vi "Sample Variance PtByPt.vi"(0 "x":dbl format="%0.2f", 1 "sample length":i32=100, 2 "initialize":bool) -> (3 "mean":dbl format="%0.2f", 4 "sample variance":dbl format="%0.2f", 5 "error":i32)   [LabVIEW 2020, in "NI_PtbyPt.lvlib"]
doc: "Computes the <B>mean</B> and <B>sample variance</B> of the values in the set of input data points specified by <B>sample length</B>."
uses:
  NI_PtbyPt.lvlib
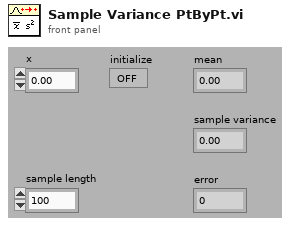
[diagram p1: front panel]
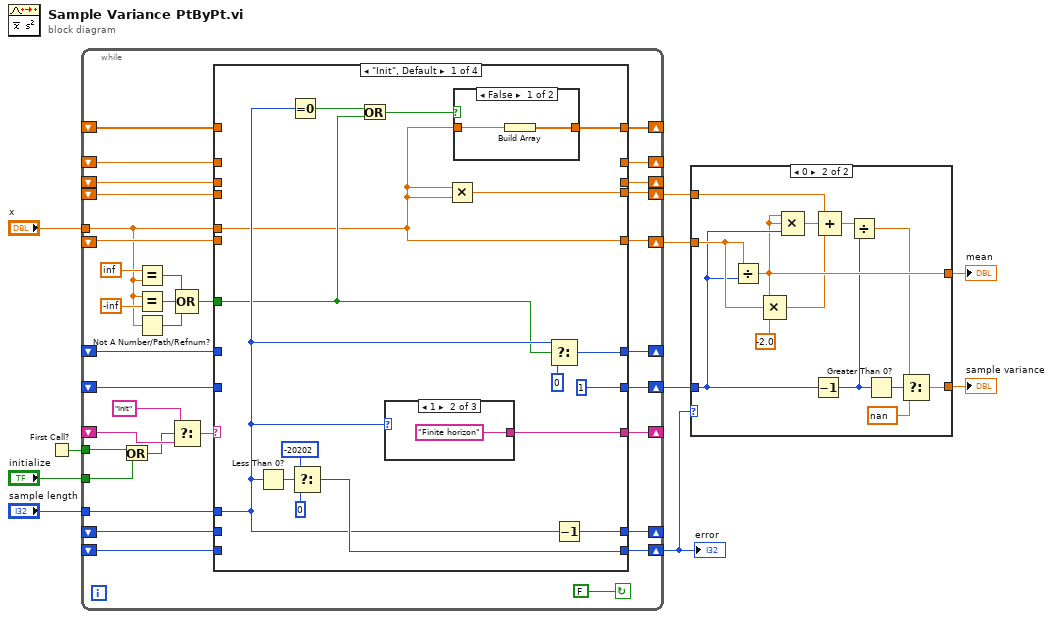
[diagram p0: block diagram]
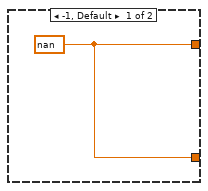
[diagram p2: hidden frame]
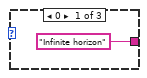
[diagram p4: hidden frame]
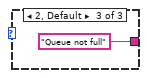
[diagram p5: hidden frame]
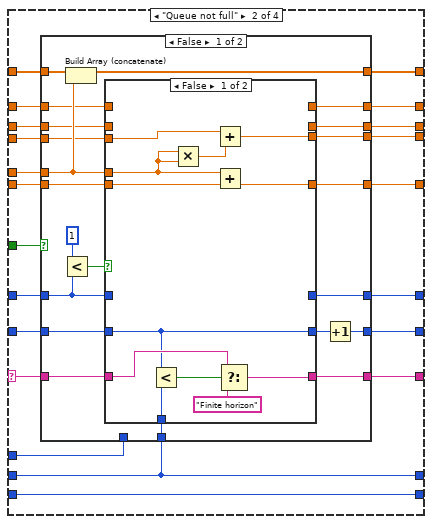
[diagram p6: hidden frame]
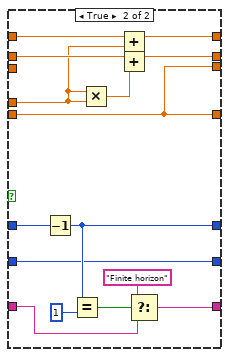
[diagram p7: hidden frame]
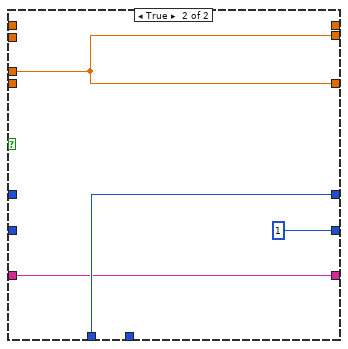
[diagram p8: hidden frame]
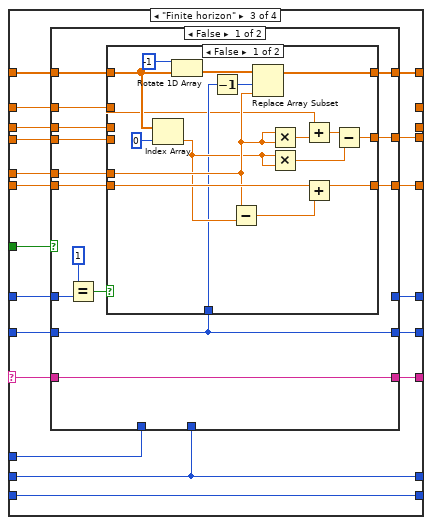
[diagram p9: hidden frame]
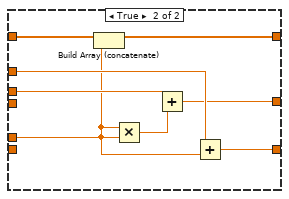
[diagram p10: hidden frame]
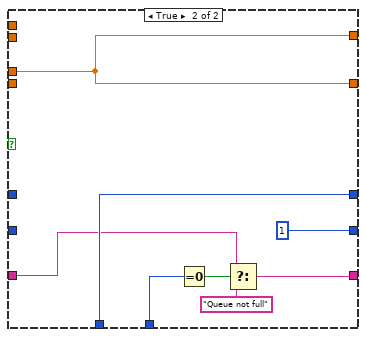
[diagram p11: hidden frame]
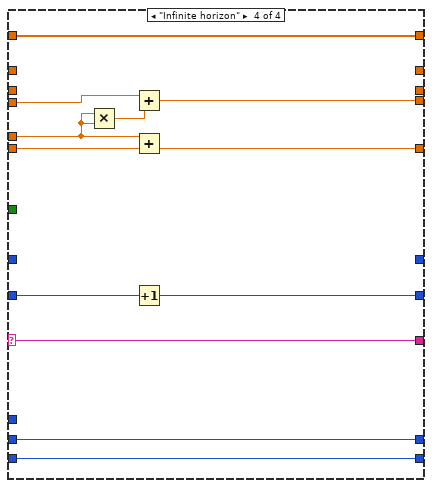
[diagram p12: hidden frame]
diagram:
  n1 = First Call?() -> (First Call?: T/F=w6:bool)
  n2 = while {
    tunnel: w6 -> [w29]
    shift-left: _ -> [w32]
    shift-right: [w31] -> _
    shift-left: _ -> [w33]
    shift-right: [w34] -> w9
    shift-left: _ -> [w36]
    shift-right: [w35] -> _
    shift-left: _ -> [w38]
    shift-right: [w39] -> w8
    shift-left: _ -> [w40]
    shift-right: [w41] -> w10
    shift-left: _ -> [w44]
    shift-right: [w37] -> _
    shift-right: [w21] -> _
    shift-left: _ -> [w16]
    shift-right: [w20] -> _
    shift-left: _ -> [w19]
    shift-right: [w18] -> _
    shift-left: _ -> [w17]
    shift-right: [w15] -> w5
    shift-left: _ -> [w14]
    tunnel: "x" -> [w13]
    tunnel: "sample length" -> [w12]
    tunnel: "initialize" -> [w11]
    stop <- FALSE continue-if-true
    n3 = Or(x=w29, y=w11) -> (x .or. y?=w28:bool)
    n4 = Equal?(x=inf, y=w13) -> (x = y?=w24:bool)
    n5 = Equal?(x=w13, y=-inf) -> (x = y?=w25:bool)
    n6 = Not A Number/Path/Refnum?(number/path/refnum=w13) -> (NaN/Path/Refnum?=w23:bool)
    n7 = Select(t="Init", s=w28, f=w44) -> (s? t:f=w42:string)
    n8 = Compound Arithmetic op=OR(w24, w25, w23) -> (w22:bool)
    n9 = case shown="\"Init\", Default" w42 {
      selector: w42 -> [_ w82 w149 w213]
      tunnel: [w45 w84 w154 w215] -> w41
      tunnel: w40 -> [_ w78 w151 w216]
      tunnel: w13 -> [w45 w80 w150 w209]
      tunnel: [1 w67 w147 w205] -> w39
      tunnel: w38 -> [_ w83 w157 w214]
      tunnel: [w51 w81 w148 w213] -> w37
      tunnel: w36 -> [_ w86 w155 w212]
      tunnel: [w46 w85 w156 w212] -> w35
      tunnel: w12 -> [w50 w68 w142 _]
      tunnel: [w56 w79 w152 w208] -> w34
      tunnel: w33 -> [_ w77 w153 w211]
      tunnel: [w55 w76 w140 w207] -> w31
      tunnel: w32 -> [_ w76 w140 w207]
      tunnel: w22 -> [w48 w75 w146 _]
      tunnel: [w53 w69 w141 _] -> w21
      tunnel: [_ w74 _ _] -> w20
      tunnel: w19 -> [_ w73 w143 _]
      tunnel: [_ w72 _ _] -> w18
      tunnel: w17 -> [_ w71 w144 _]
      tunnel: w16 -> [_ w70 w145 _]
      tunnel: [w52 w66 w139 w206] -> w15
      tunnel: w14 -> [_ w66 w139 w206]
      frame "Init", Default {
        n10 = Less Than 0?(x=w50) -> (x < 0?=w57:bool)
        n11 = Equal To 0?(x=w50) -> (x = 0?=w49:bool)
        n12 = Select(t=-20202, s=w57, f=0) -> (s? t:f=w52:i32)
        n13 = Or(x=w49, y=w48) -> (x .or. y?=w47:bool)
        n14 = case shown="1" w50 {
          tunnel: ["Infinite horizon" "Finite horizon" "Queue not full" ("f")] -> w51
          frame 0 {
          }
          frame 1 {
          }
          frame 2, Default {
          }
        }
        n15 = Multiply(x=w45, y=w45) -> (x*y=w56:dbl)
        n16 = case shown="False" w47 {
          tunnel: [w62 _] -> w46
          tunnel: w45 -> [w61 _]
          frame False {
            n17 = Build Array(w61) -> (w62:dbl[])
          }
          frame True {
          }
        }
        n18 = Select(t=w50, s=w48, f=0) -> (s? t:f=w53:i32)
        n19 = Decrement(x=w50) -> (x-1=w55:i32)
      }
      frame "Queue not full" {
        n20 = case shown="False" w75 {
          tunnel: w86 -> [w107 _]
          tunnel: [w106 _] -> w85
          tunnel: [w105 w135] -> w84
          tunnel: w83 -> [w97 _]
          tunnel: w82 -> [w104 w136]
          tunnel: [w103 w136] -> w81
          tunnel: w80 -> [w102 w135]
          tunnel: [w101 w135] -> w79
          tunnel: w78 -> [w100 _]
          tunnel: w77 -> [w99 _]
          tunnel: w76 -> [w98 _]
          tunnel: [w90 1] -> w67
          tunnel: [w95 _] -> w74
          tunnel: w73 -> [w94 _]
          tunnel: [w93 _] -> w72
          tunnel: w71 -> [w92 _]
          tunnel: w70 -> [w87 _]
          tunnel: [w91 w138] -> w69
          tunnel: w68 -> [_ w138]
          frame False {
            n21 = Less?(x=1, y=w87) -> (x < y?=w88:bool)
            n22 = Build Array (concatenate)(w107, w102) -> (w106:dbl[])
            n23 = case shown="False" w88 {
              tunnel: [w119 w128] -> w105
              tunnel: w104 -> [w117 w120]
              tunnel: [w115 w121] -> w103
              tunnel: w102 -> [w114 w131]
              tunnel: [w113 w128] -> w101
              tunnel: w100 -> [w112 w128]
              tunnel: w99 -> [w111 _]
              tunnel: w98 -> [w109 _]
              tunnel: w97 -> [w108 w122]
              tunnel: [w108 w122] -> w96
              tunnel: [_ w133] -> w95
              tunnel: w94 -> [_ w132]
              tunnel: [_ w130] -> w93
              tunnel: w92 -> [_ w129]
              tunnel: w87 -> [_ w124]
              tunnel: [_ w123] -> w91
              frame False {
                n24 = Less?(x=w108, y=w109) -> (x < y?=w118:bool)
                n25 = Multiply(x=w114, y=w114) -> (x*y=w110:dbl)
                n26 = Add(x=w111, y=w110) -> (x+y=w113:dbl)
                n27 = Add(x=w114, y=w112) -> (x+y=w119:dbl)
                n28 = Select(t=w117, s=w118, f="Finite horizon") -> (s? t:f=w115:string)
              }
              frame True {
                n29 = Decrement(x=w124) -> (x-1=w123:i32)
                n30 = Equal?(x=w123, y=1) -> (x = y?=w127:bool)
                n31 = Multiply(x=w131, y=w131) -> (x*y=w134:dbl)
                n32 = Add(x=w129, y=w131) -> (x+y=w130:dbl)
                n33 = Add(x=w132, y=w134) -> (x+y=w133:dbl)
                n34 = Select(t="Finite horizon" ("f"), s=w127, f=w120) -> (s? t:f=w121:string)
              }
            }
            n35 = Increment(x=w96) -> (x+1=w90:i32)
          }
          frame True {
          }
        }
      }
      frame "Finite horizon" {
        n36 = case shown="False" w146 {
          tunnel: w157 -> [w163 _]
          tunnel: [w171 _] -> w156
          tunnel: w155 -> [w170 _]
          tunnel: [w169 w197] -> w154
          tunnel: w153 -> [w168 _]
          tunnel: [w167 w197] -> w152
          tunnel: w151 -> [w166 _]
          tunnel: w150 -> [w165 w197]
          tunnel: w149 -> [w164 w198]
          tunnel: [w164 w200] -> w148
          tunnel: [w163 1] -> w147
          tunnel: w145 -> [w161 _]
          tunnel: w144 -> [w159 _]
          tunnel: w143 -> [w158 _]
          tunnel: w142 -> [_ w204]
          tunnel: [_ w204] -> w141
          tunnel: w140 -> [_ w199]
          frame False {
            n37 = Equal?(x=1, y=w161) -> (x = y?=w160:bool)
            n38 = case shown="False" w160 {
              tunnel: [w184 w191] -> w171
              tunnel: w170 -> [w183 w195]
              tunnel: [w182 w189] -> w169
              tunnel: w168 -> [w172 _]
              tunnel: [w178 w190] -> w167
              tunnel: w166 -> [w177 _]
              tunnel: w165 -> [w176 w192]
              tunnel: w163 -> [w173 _]
              tunnel: w159 -> [_ w194]
              tunnel: w158 -> [_ w193]
              frame False {
                n39 = Index Array(array=w183, index=0 ("Index")) -> (element=w175:dbl)
                n40 = Rotate 1D Array(1:w183, 2:i16 -1 ("n")) -> (0:w186:dbl[])
                n41 = Decrement(x=w173) -> (x-1=w185:i32)
                n42 = Subtract(x=w176, y=w175) -> (x-y=w174:dbl)
                n43 = Replace Array Subset(array=w186, new element=w176, index=w185) -> (w184:dbl[])
                n44 = Multiply(x=w176, y=w176) -> (x*y=w181:dbl)
                n45 = Multiply(x=w175, y=w175) -> (x*y=w179:dbl)
                n46 = Add(x=w172, y=w181) -> (x+y=w180:dbl)
                n47 = Add(x=w177, y=w174) -> (x+y=w182:dbl)
                n48 = Subtract(x=w180, y=w179) -> (x-y=w178:dbl)
              }
              frame True {
                n49 = Build Array (concatenate)(w195, w192) -> (w191:dbl[])
                n50 = Multiply(x=w192, y=w192) -> (x*y=w196:dbl)
                n51 = Add(x=w193, y=w196) -> (x+y=w190:dbl)
                n52 = Add(x=w194, y=w192) -> (x+y=w189:dbl)
              }
            }
          }
          frame True {
            n53 = Equal To 0?(x=w199) -> (x = 0?=w203:bool)
            n54 = Select(t=w198, s=w203, f="Queue not full") -> (s? t:f=w200:string)
          }
        }
      }
      frame "Infinite horizon" {
        n55 = Multiply(x=w209, y=w209) -> (x*y=w210:dbl)
        n56 = Add(x=w211, y=w210) -> (x+y=w208:dbl)
        n57 = Add(x=w209, y=w216) -> (x+y=w215:dbl)
        n58 = Increment(x=w214) -> (x+1=w205:i32)
      }
    }
  }
  "error" <- w5
  n59 = case shown="0" w5 {
    tunnel: w10 -> [_ w230]
    tunnel: w9 -> [_ w228]
    tunnel: w8 -> [_ w225]
    tunnel: [w217 w224] -> w7
    tunnel: [w217 w218] -> w1
    frame -1, Default {
      w217 = nan
    }
    frame 0 {
      n60 = Divide(x=w230, y=w225) -> (x/y=w224:dbl)
      n61 = Compound Arithmetic op=MULTIPLY(w224, w230, -2.0) -> (w223:dbl)
      n62 = Compound Arithmetic op=MULTIPLY(w224, w224, w225) -> (w227:dbl)
      n63 = Decrement(x=w225) -> (x-1=w222:i32)
      n64 = Compound Arithmetic op=ADD(w228, w227, w223) -> (w226:dbl)
      n65 = Divide(x=w226, y=w222) -> (x/y=w220:dbl)
      n66 = Greater Than 0?(x=w222) -> (x > 0?=w221:bool)
      n67 = Select(t=w220, s=w221, f=nan) -> (s? t:f=w218:dbl)
    }
  }
  "mean" <- w7
  "sample variance" <- w1
